vi "TypeConv_Register Existing Complex Types.vi"(4 "Manifestation Ancestors":T1, 10 "Module Root Dir":path, 11 "Type Categories":T2) -> (3 "Type Categories Dup":T2)   [LabVIEW 2013]
uses:
  Data Structures/JSON/Type Categories.ctl
  Data Structures/JSON/TypeConv.ctl
  Data Structures/JSON/Simple Struct.ctl
  Data Structures/JSON/Param.ctl
  Data Structures/JSON/Method.ctl
  Data Structures/JSON/Class.ctl
  Data Structures/JSON/Enum.ctl
  Data Structures/JSON/Enum Value.ctl
  Data Structures/JSON/Property.ctl
  Data Structures/Manifestation Ancestors.ctl
  Category.ctl
  Action.ctl
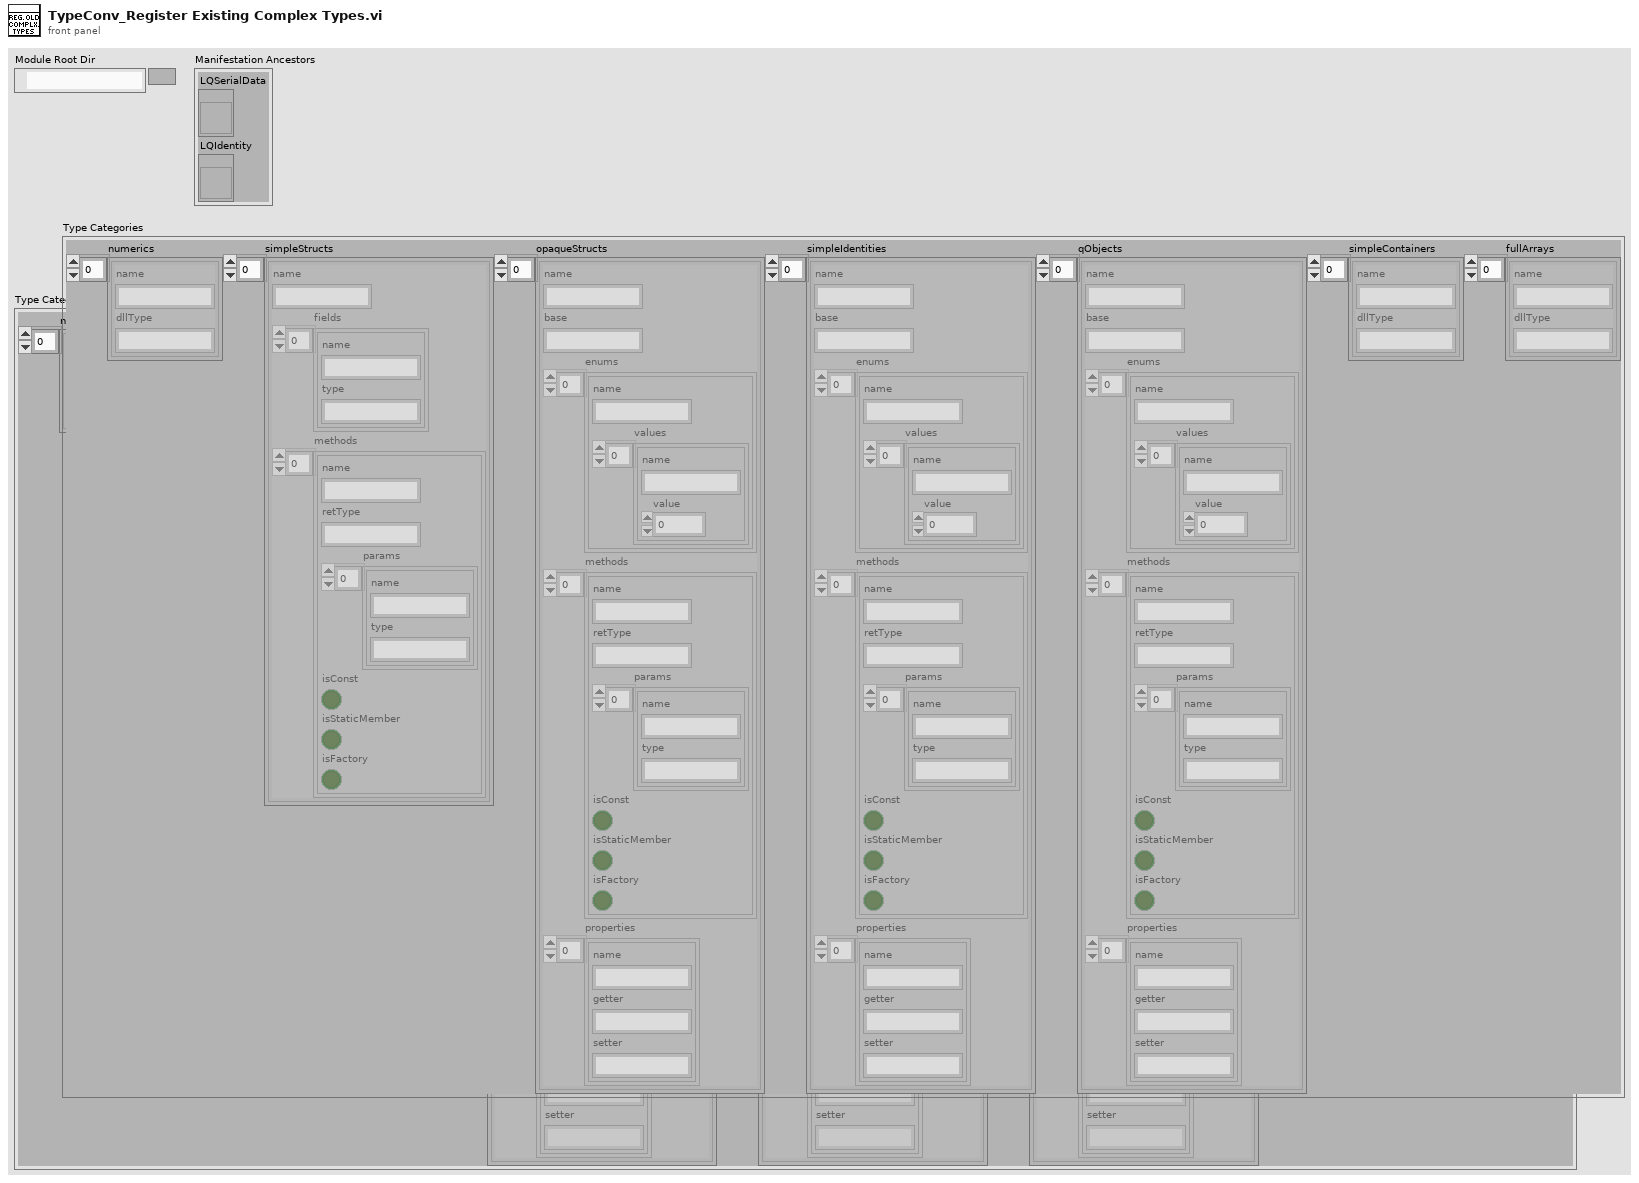
[diagram p1: front panel]
types:
  T1 = typedef "Manifestation Ancestors.ctl" = cluster{"LQSerialData":refnum<vi>, "LQIdentity":refnum<vi>}
  T2 = typedef "Type Categories.ctl" = cluster{"numerics":T3[], "simpleStructs":T4[], "opaqueStructs":T7[], "simpleIdentities":T7[], "qObjects":T7[], "simpleContainers":T3[], "fullArrays":T3[]}
  T3 = typedef "TypeConv.ctl" = cluster{"name":string, "dllType":string}
  T4 = typedef "Simple Struct.ctl" = cluster{"name":string, "fields":T5[], "methods":T6[]}
  T5 = typedef "Param.ctl" = cluster{"name":string, "type":string}
  T6 = typedef "Method.ctl" = cluster{"name":string, "retType":string, "params":T5[], "isConst":bool, "isStaticMember":bool, "isFactory":bool}
  T7 = typedef "Class.ctl" = cluster{"name":string, "base":string, "enums":T8[], "methods":T6[], "properties":T10[]}
  T8 = typedef "Enum.ctl" = cluster{"name":string, "values":T9[]}
  T9 = typedef "Enum Value.ctl" = cluster{"name":string, "value":i32}
  T10 = typedef "Property.ctl" = cluster{"name":string, "getter":string, "setter":string}
  T11 = typedef "Category.ctl" = enum16{"Invalid", "Void", "Boolean", "Numeric", "Enum", "SimpleStruct", "OpaqueStruct", "SimpleIdentity", "QObject", "SimpleContainer", "FullArray"}
  T12 = typedef "Action.ctl" = enum16{"Register Type", "Register Projection", "Obtain Writer", "Get Projection", "Get Type Path"}
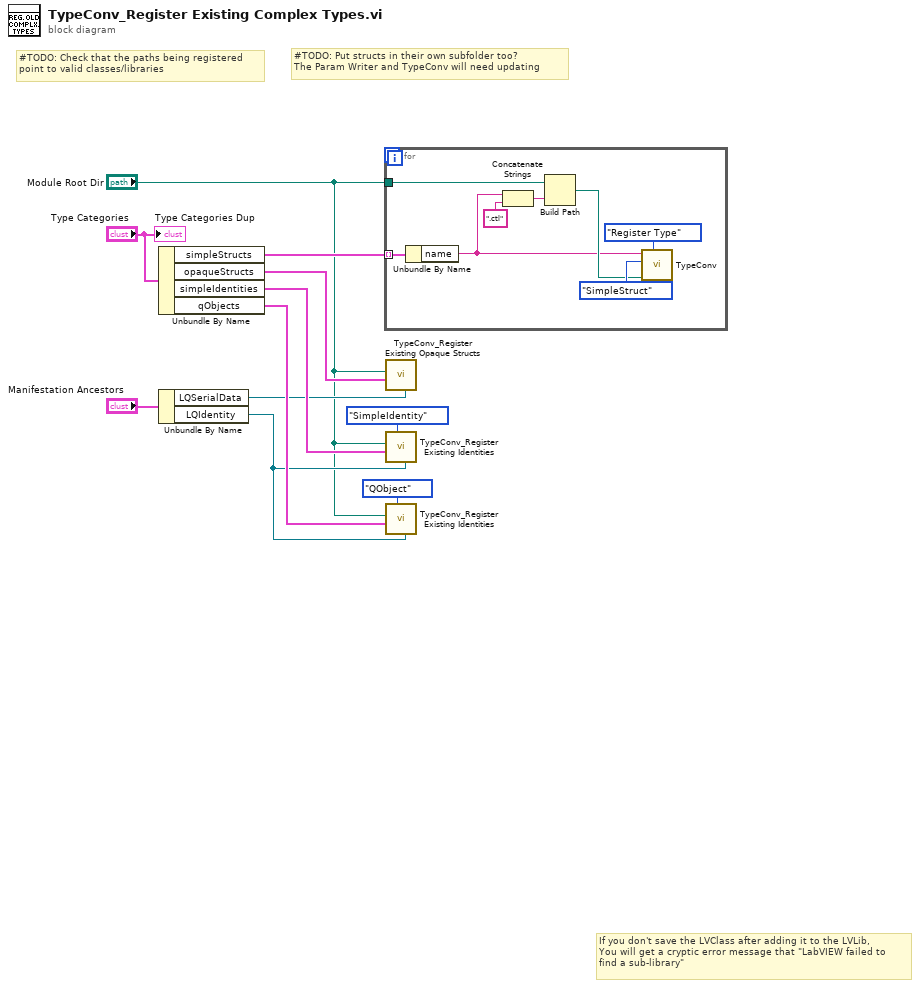
[diagram p0: block diagram]
diagram:
  # "#TODO: Check that the paths being registered\npoint to valid classes/libraries"
  # "If you don't save the LVClass after adding it to the LVLib,\nYou will get a cryptic error message that \"LabVIEW failed to\nfind a sub-library\""
  # "#TODO: Put structs in their own subfolder too?\nThe Param Writer and TypeConv will need updating"
  n1 = Unbundle By Name("Type Categories") -> ("simpleStructs"=w10:T4[], "opaqueStructs"=w7:T7[], "simpleIdentities"=w9:T7[], "qObjects"=w8:T7[])
  n2 = Unbundle By Name("Manifestation Ancestors") -> ("LQSerialData"=w5:refnum<vi>, "LQIdentity"=w4:refnum<vi>)
  n3 = for {
    tunnel: w10 -> [w19] mode=indexing
    tunnel: "Module Root Dir" -> [w18]
    n4 = Unbundle By Name(w19) -> ("name"=w12:string)
    n5 = Concatenate Strings(w12, ".ctl" ("string")) -> (w16:string)
    n6 = Build Path(base path=w18, name or relative path=w16) -> (appended path=w13:path)
    n7 = call "TypeConv.vi"("Action"=Action."Register Type", "Type Path"=w13, "Category"=Category."SimpleStruct", "Type Name"=w12) -> ()  [unwired: 4 in, 4 out]
  }
  n8 = call "TypeConv_Register Existing Opaque Structs.vi"("Manifestation Ancestor"=w5, "Classes"=w7, "Module Root Dir"="Module Root Dir") -> ()  [unwired: 9 in]
  n9 = call "TypeConv_Register Existing Identities.vi"("Manifestation Ancestor"=w4, "Category"=Category."SimpleIdentity", "Classes"=w9, "Module Root Dir"="Module Root Dir") -> ()  [unwired: 8 in]
  n10 = call "TypeConv_Register Existing Identities.vi"("Manifestation Ancestor"=w4, "Category"=Category."QObject", "Classes"=w8, "Module Root Dir"="Module Root Dir") -> ()  [unwired: 8 in]
  "Type Categories Dup" <- "Type Categories"
